vi "StateMachineSubpanel.vi"() -> ()   [LabVIEW 2016]
uses:
  Controls/Config.ctl
  Utilities/DataShare/DataShare.lvclass
  Controls/DAQ.ctl
  Utilities/ControlValues/ControlValues.lvclass
  <vilib>/Utility/error.llb/DialogType.ctl
panel:
  in  "SelectPanel":i32(listbox)=-1
  out "Status":string
  # "Logo"
  # "Blank area for constantly available displays"
  # "Blank area for constantly\navailable displays"
  # "Blank area for constantly available displays, delete splitter if not needed"
  # "Blank area for constantly available displays"
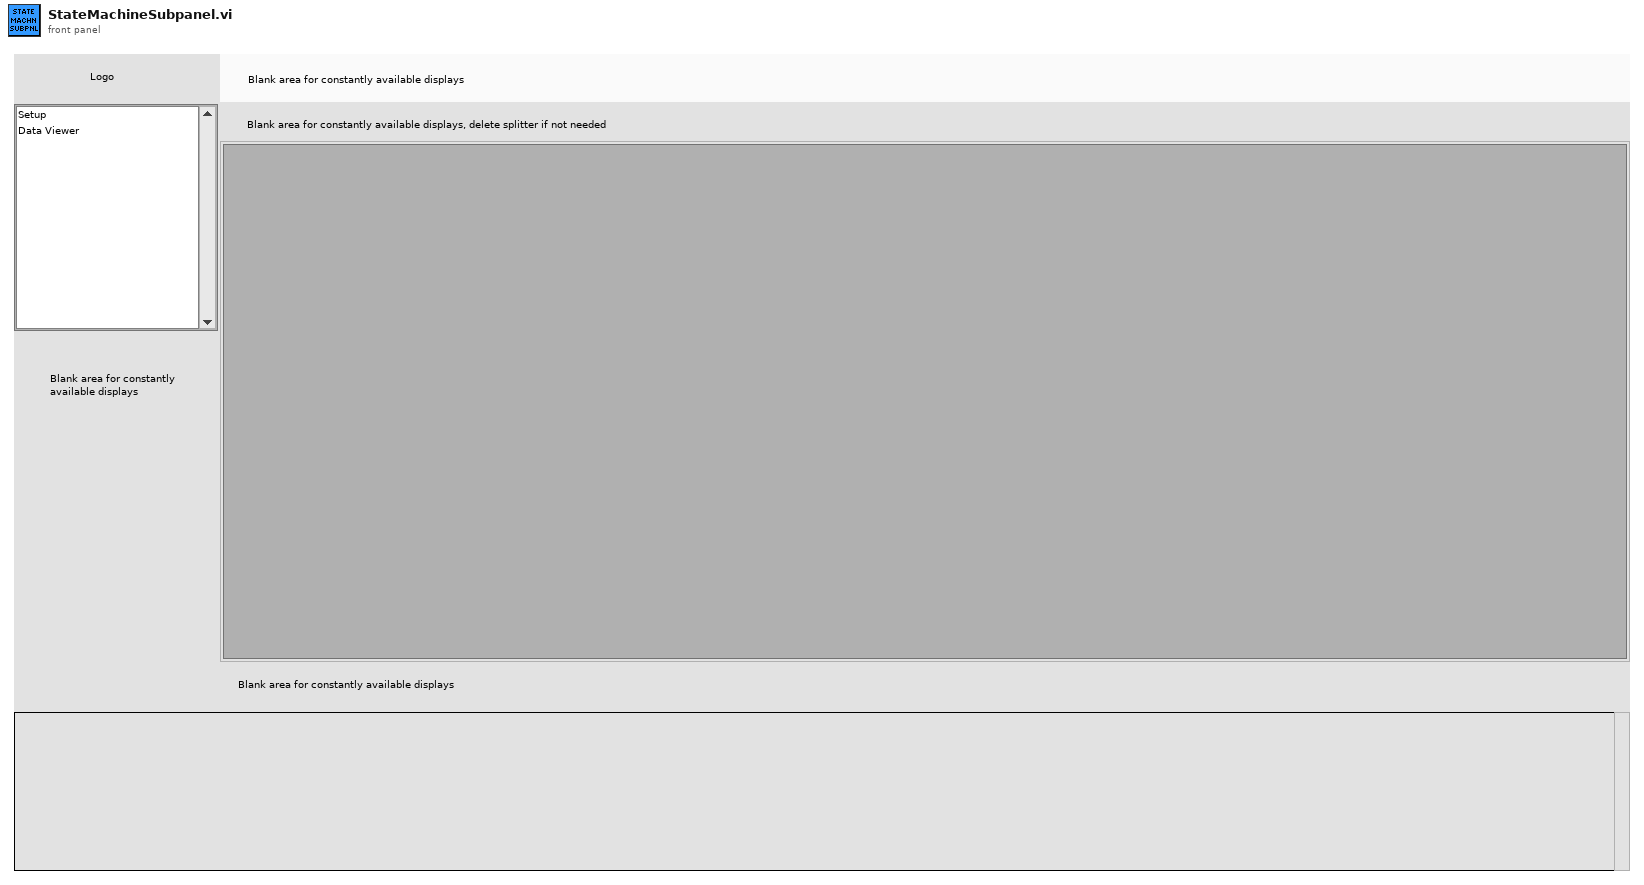
[diagram p1: front panel]
types:
  T1 = typedef "Config.ctl" = cluster{"Subpanels":cluster{"Name":string, "Pathname":string}[], "DAQ":cluster{"Name":string, "Value":string}[]}
  T2 = cluster{"Error":errorcluster, "SubpanelRefs":refnum<vi>[], "SubpanelRef":refnum<vi>, "ControlValues":refnum<class "ControlValues.lvclass">, "AppKind":enum32{"invalid app kind", "Development System", "Run Time System", "Student Edition", "Embedded LabVIEW", "Evaluation", "Custom"}, "LogFolder":path, "ConfigFolder":path, "Config":T1}
  T3 = enum32{"invalid app kind", "Development System", "Run Time System", "Student Edition", "Embedded LabVIEW", "Evaluation", "Custom"}
  T4 = typedef "DialogType.ctl" = u16
  T5 = cluster{"Error":errorcluster, "Config":T1, "Names":string[], "Values":dbl[], "DataShare":refnum<class "DataShare.lvclass">}
  T6 = typedef "DAQ.ctl" = cluster{"Names":string[], "Values":dbl[]}
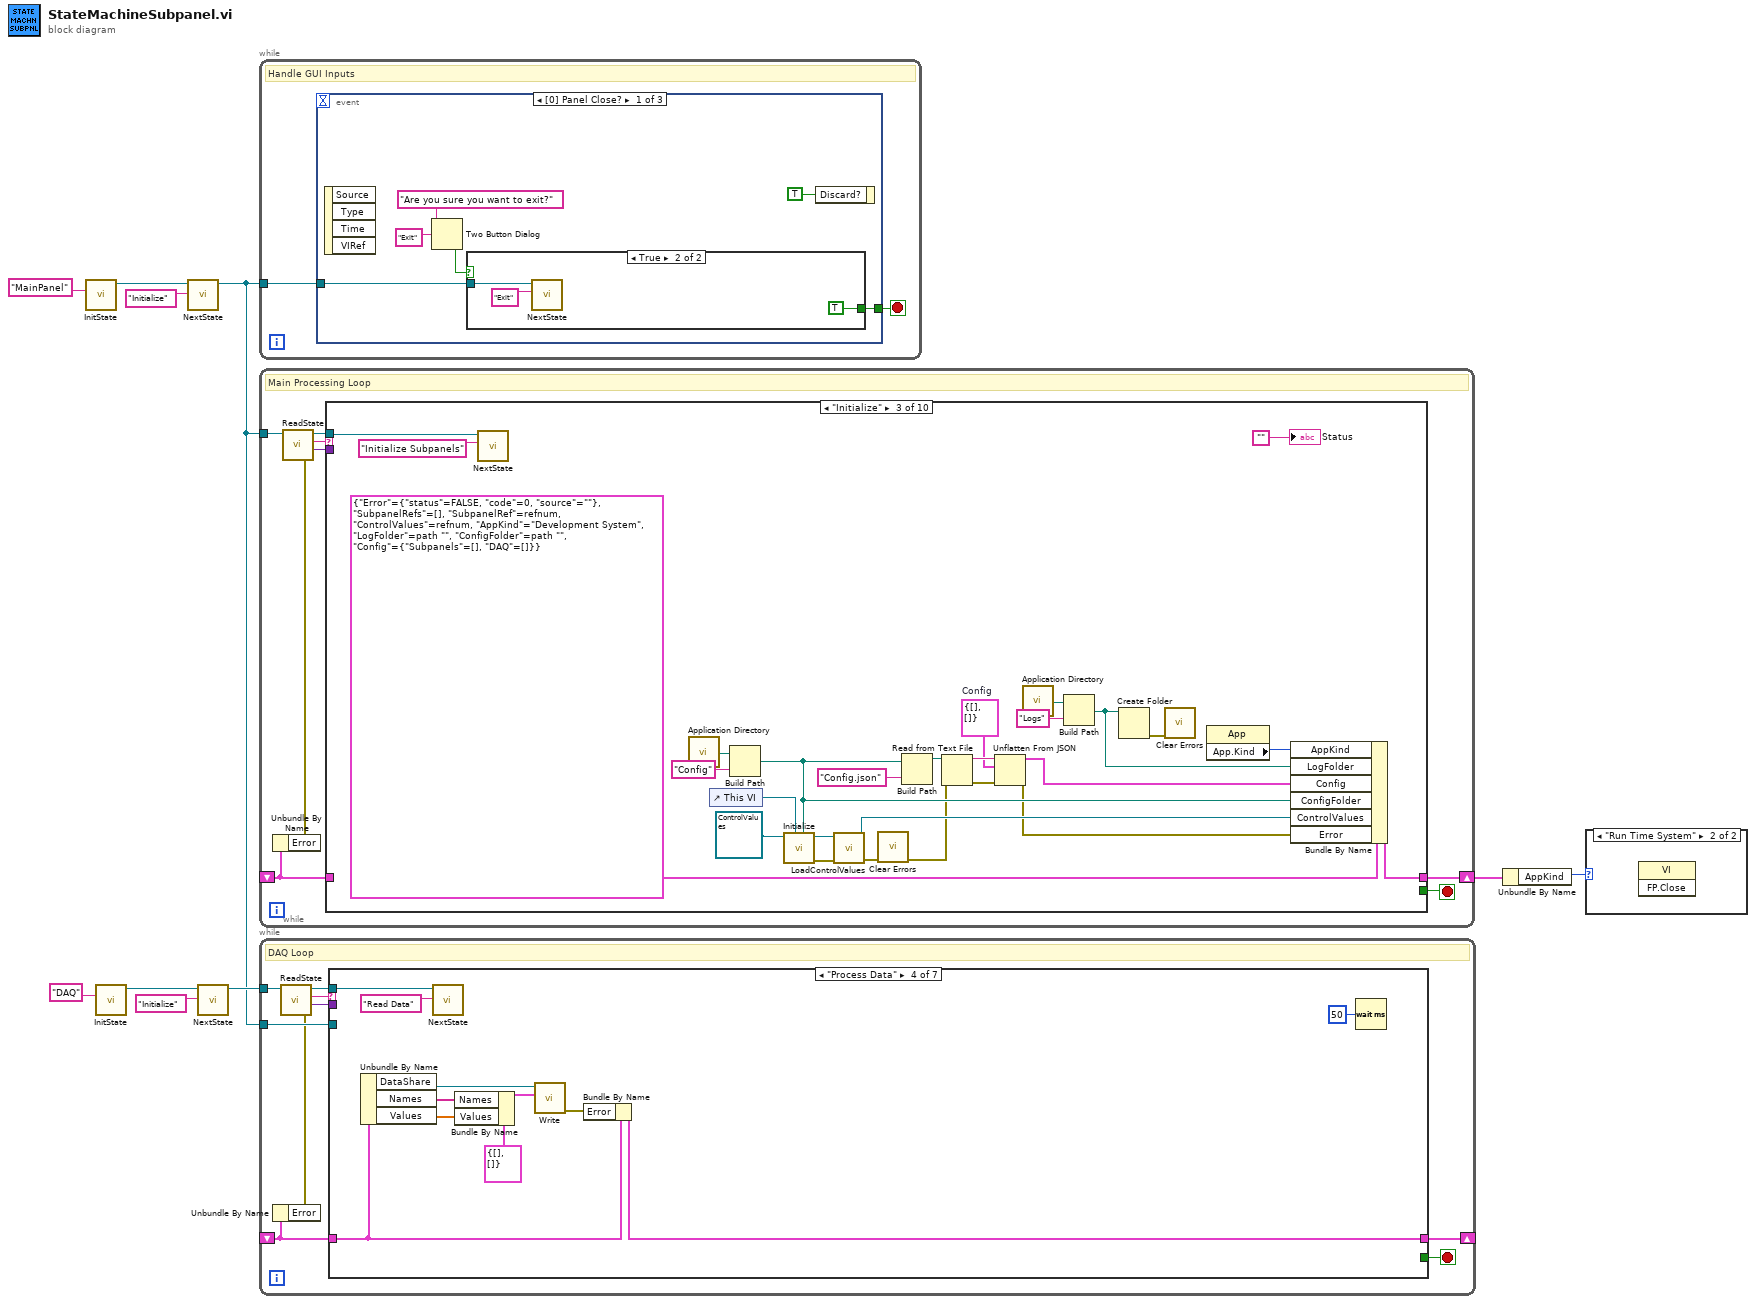
[diagram p0: block diagram]
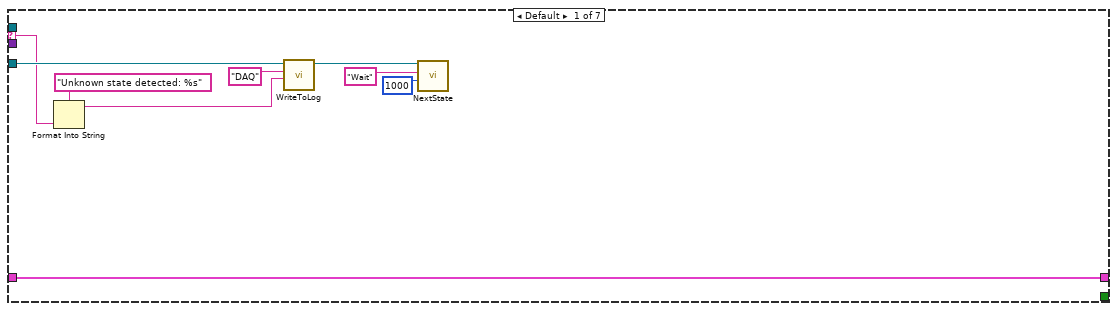
[diagram p2: hidden frame]
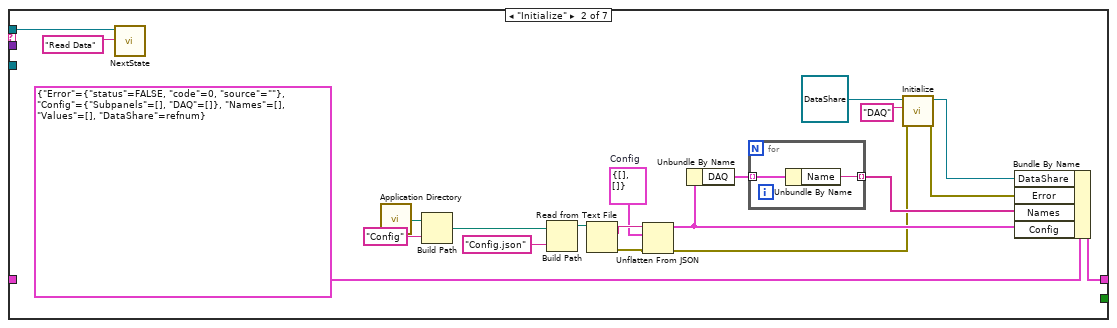
[diagram p3: hidden frame]
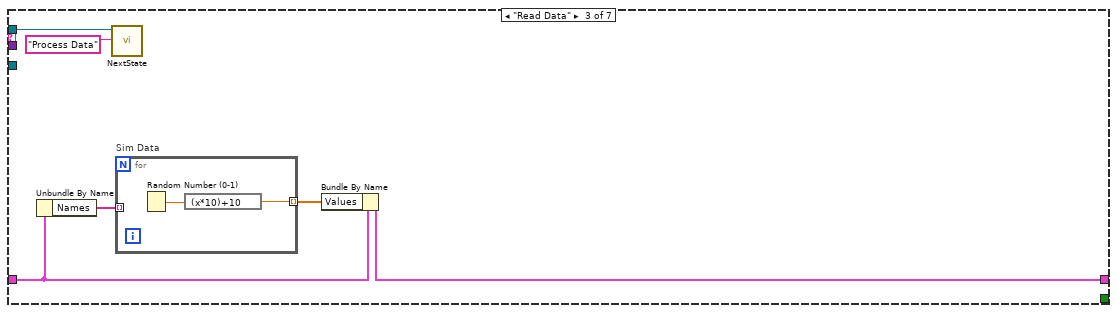
[diagram p4: hidden frame]
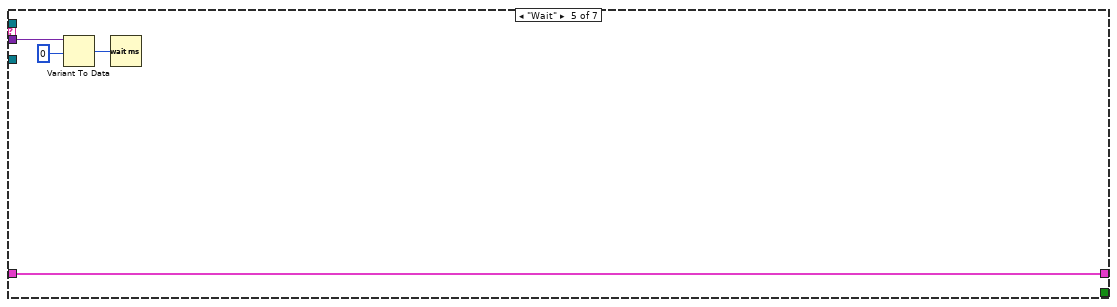
[diagram p5: hidden frame]
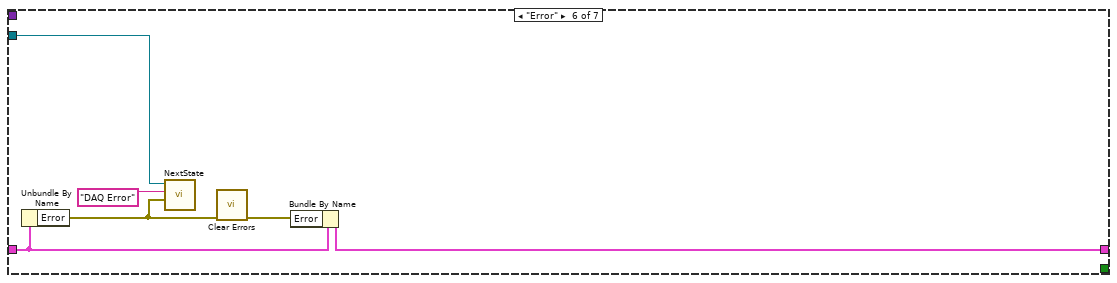
[diagram p6: hidden frame]
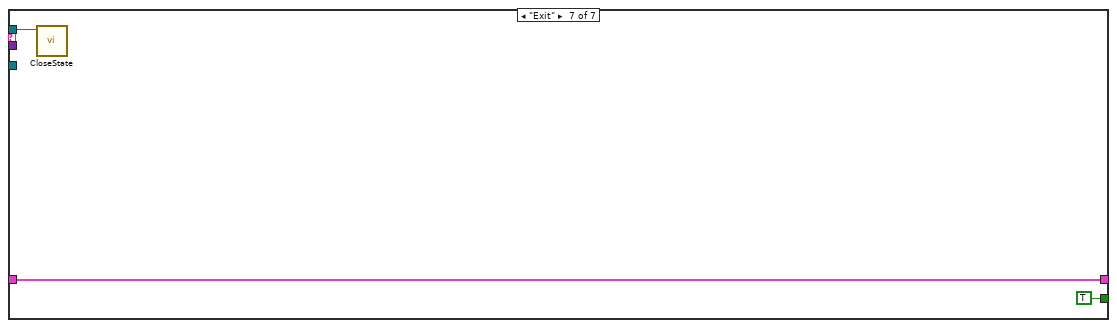
[diagram p7: hidden frame]
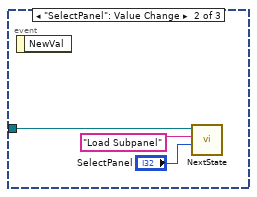
[diagram p10: hidden frame]
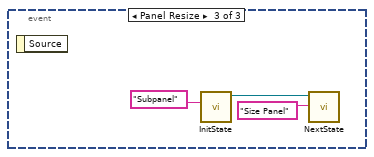
[diagram p11: hidden frame]
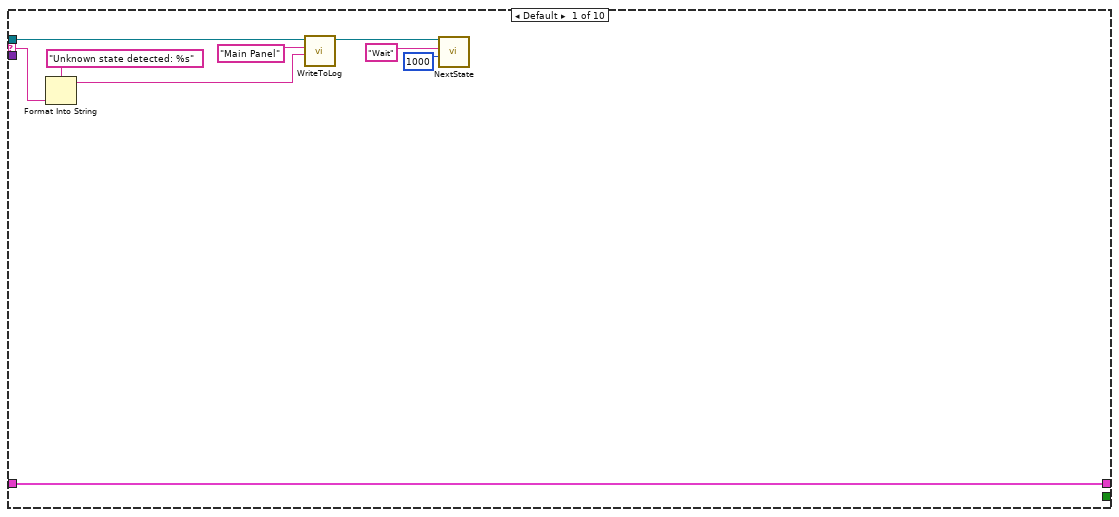
[diagram p12: hidden frame]
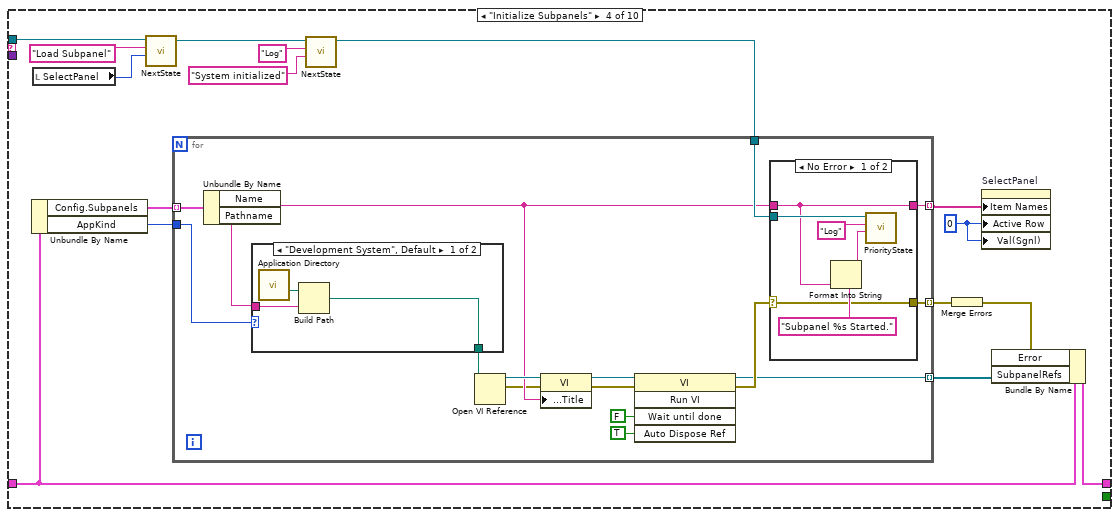
[diagram p14: hidden frame]
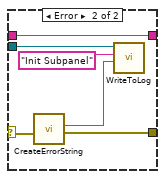
[diagram p15: hidden frame]
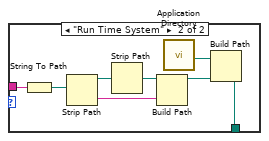
[diagram p16: hidden frame]
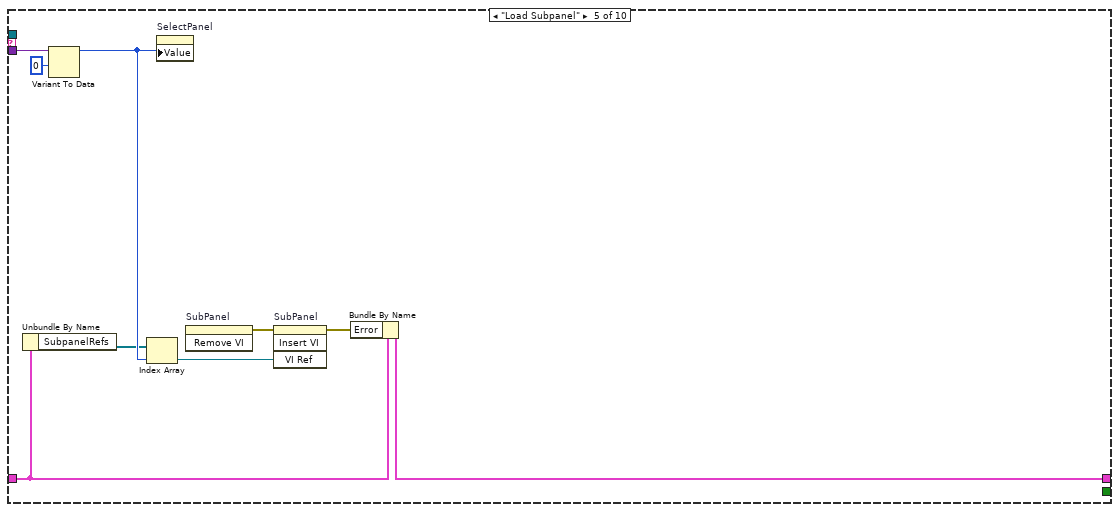
[diagram p17: hidden frame]
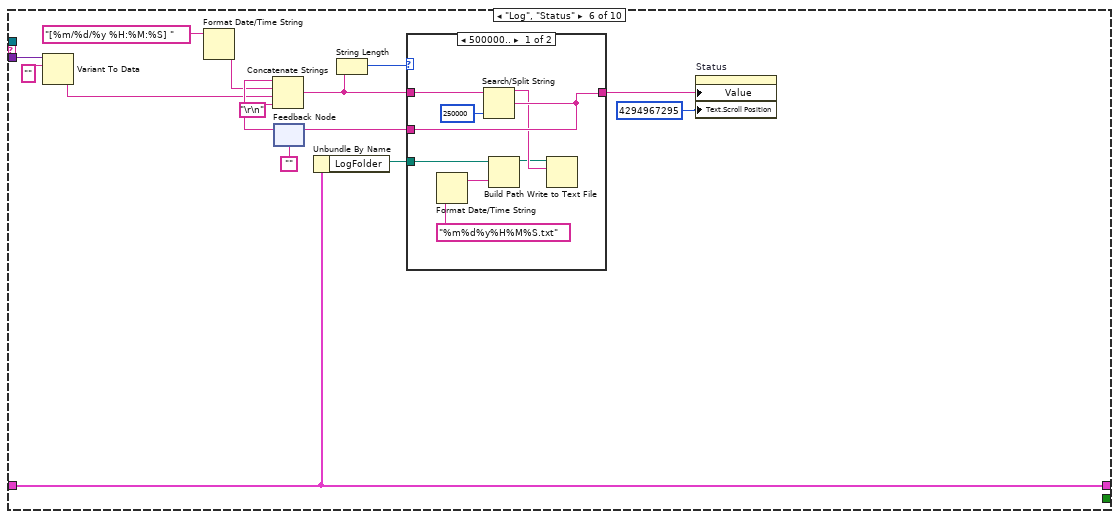
[diagram p18: hidden frame]
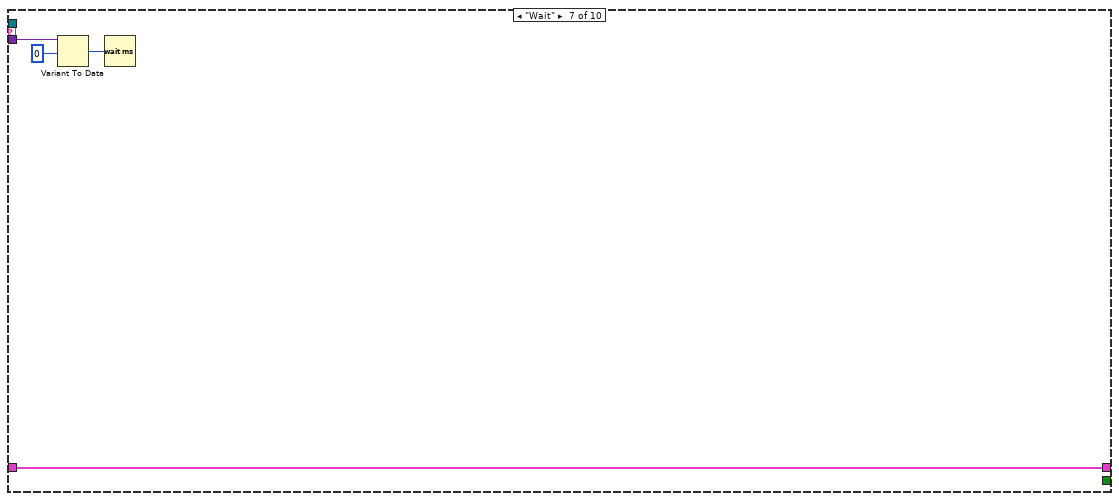
[diagram p20: hidden frame]
diagram:
  n1 = call "InitState.vi"("Name"="MainPanel" ("name (unnamed)")) -> ("Queue Out"=w6:refnum<queue>)  [unwired: 8 in, 1 out]
  n2 = call "InitState.vi"("Name"="DAQ" ("name (unnamed)")) -> ("Queue Out"=w3:refnum<queue>)  [unwired: 8 in, 1 out]
  n3 = call "NextState.vi"("State"="Initialize" ("element"), "Queue In"=w6) -> ("Queue Out"=w1:refnum<queue>)  [unwired: 8 in, 1 out]
  n4 = call "NextState.vi"("State"="Initialize" ("element"), "Queue In"=w3) -> ("Queue Out"=w2:refnum<queue>)  [unwired: 8 in, 1 out]
  n5 = while {
    tunnel: w1 -> [w12]
    stop <- w11 stop-if-true
    # "Handle GUI Inputs"
    n6 = event shown="[0] Panel Close?" {
      selector: _ -> [_ _ _]
      dyn-events: _ -> [_ _ _]
      timeout: _ -> [_ _ _]
      tunnel: w12 -> [w18 w23 _]
      tunnel: [w13 _ _] -> w11
      event Panel Close? {
        n7 = event-data() -> ()  [unwired: 1 in, 4 out]
        n8 = Two Button Dialog(message="Are you sure you want to exit?", 2:"Exit" ("T button name (\"OK\")")) -> (T button?=w14:bool)  [unwired: 1 in]
        n9 = case shown="True" w14 {
          tunnel: w18 -> [_ w19]
          tunnel: [_ TRUE] -> w13
          frame False {
          }
          frame True {
            n10 = call "NextState.vi"("State"="Exit" ("element"), "Queue In"=w19) -> ()  [unwired: 8 in, 2 out]
          }
        }
        n11 = event-data("Discard?"=TRUE) -> ()  [unwired: 1 in, 1 out]
      }
      event "SelectPanel": Value Change {
        n12 = event-data() -> ()  [unwired: 1 in, 1 out]
        n13 = call "NextState.vi"("Data"="SelectPanel", "State"="Load Subpanel", "Queue In"=w23) -> ()  [unwired: 7 in, 2 out]
      }
      event Panel Resize {
        n14 = event-data() -> ()  [unwired: 1 in, 1 out]
        n15 = call "InitState.vi"("Name"="Subpanel" ("name (unnamed)")) -> ("Queue Out"=w25:refnum<queue>)  [unwired: 8 in, 1 out]
        n16 = call "NextState.vi"("State"="Size Panel" ("element"), "Queue In"=w25) -> ()  [unwired: 8 in, 2 out]
      }
    }
  }
  n17 = while {
    tunnel: w1 -> [w33]
    shift-right: [w35] -> w10
    shift-left: _ -> [w29]
    stop <- w34 stop-if-true
    # "Main Processing Loop"
    n18 = Unbundle By Name(w29) -> ("Error"=w28:errorcluster)
    n19 = call "ReadState.vi"("Error In"=w28, "Queue In"=w33) -> ("Data"=w30:variant, "State"=w31:string, "Queue Out"=w32:refnum<queue>)  [unwired: 6 in, 1 out]
    n20 = case shown="\"Initialize\"" w31 {
      tunnel: w32 -> [w41 _ w47 w79 _ _ _ w181 w205 _]
      tunnel: w30 -> [_ _ _ _ w135 w151 w164 w167 _ _]
      selector: w31 -> [w43 _ _ _ _ _ _ w168 _ _]
      tunnel: [w42 w45 w72 w75 w133 w138 w161 w183 w204 w215] -> w35
      tunnel: [_ _ _ _ _ _ _ _ TRUE _] -> w34
      tunnel: w29 -> [w42 w45 _ w76 w132 w138 w161 w166 w204 w215]
      frame Default {
        n21 = Format Into String(format string="Unknown state detected: %s", w43) -> (resulting string=w36:string)  [unwired: 2 in, 1 out]
        n22 = call "WriteToLog.vi"("Data"=w36, "Source"="Main Panel", "Queue In"=w41) -> ("Queue Out"=w40:refnum<queue>)  [unwired: 7 in, 1 out]
        n23 = call "NextState.vi"("Data"=u32 1000, "State"="Wait", "Queue In"=w40) -> ()  [unwired: 7 in, 2 out]
      }
      frame "--- System ---" {
      }
      frame "Initialize" {
        w51 = T1 {"Subpanels"=[], "DAQ"=[]}  # Config
        n24 = call "NextState.vi"("State"="Initialize Subpanels" ("element"), "Queue In"=w47) -> ()  [unwired: 8 in, 2 out]
        n25 = call <vilib>:"Application Directory.vi"() -> ("Application Directory"=w60:path)
        n26 = control-ref of="This VI"() -> (w67:refnum<vi>)
        n27 = Build Path(base path=w60, name or relative path="Config") -> (appended path=w55:path)
        n28 = call "Initialize.vi"("Config Path"=w55, "VI Reference"=w67, "ControlValues in"=refnum<class "ControlValues.lvclass"> refnum) -> ("error out"=w69:errorcluster, "ControlValues out"=w70:refnum<class "ControlValues.lvclass">)  [unwired: 7 in]
        n29 = call "LoadControlValues.vi"("error in"=w69, "ControlValues in"=w70) -> ("error out"=w62:errorcluster, "ControlValues out"=w68:refnum<class "ControlValues.lvclass">)  [unwired: 8 in]
        n30 = call <vilib>:"Clear Errors.vi"("error in (no error)"=w62) -> ("error out"=w52:errorcluster)  [unwired: 5 in, 1 out]
        n31 = Build Path(base path=w55, name or relative path="Config.json") -> (appended path=w56:path)
        n32 = Read from Text File(file (use dialog)=w56, error in=w52) -> (text=w57:string, error out=w58:errorcluster)  [unwired: 2 in, 2 out]
        n33 = Unflatten From JSON(JSON string=w57, type and defaults=w51, error in (no error)=w58) -> (value=w50:T1, error out=w48:errorcluster)  [unwired: 4 in]
        n34 = call <vilib>:"Application Directory.vi"() -> ("Application Directory"=w65:path)
        n35 = Build Path(base path=w65, name or relative path="Logs") -> (appended path=w54:path)
        n36 = Create Folder(path (use dialog)=w54) -> (error out=w63:errorcluster)  [unwired: 2 in, 2 out]
        n37 = call <vilib>:"Clear Errors.vi"("error in (no error)"=w63) -> ()  [unwired: 5 in, 2 out]
        n38 = property class="App"() -> ("App.Kind"=w49:T3)  [unwired: 2 in, 2 out]
        n39 = Bundle By Name(cluster=T2 {"Error"={"status"=FALSE, "code"=0, "source"=""}, "SubpanelRefs"=[], "SubpanelRef"=refnum, "ControlValues"=refnum, "AppKind"=enum."Development System", "LogFolder"=path "", "ConfigFolder"=path "", "Config"={"Subpanels"=[], "DAQ"=[]}}, "AppKind"=w49, "LogFolder"=w54, "Config"=w50, "ConfigFolder"=w55, "ControlValues"=w68, "Error"=w48) -> (w72:T2)
        "Status" <- ""
      }
      frame "Initialize Subpanels" {
        w86 = 0 ("Active Row:Active Row Number")
        n40 = Unbundle By Name(w76) -> ("Config.Subpanels"=w88:cluster{"Name":string, "Pathname":string}[], "AppKind"=w87:T3)
        n41 = local read "SelectPanel"() -> (w83:i32)
        n42 = call "NextState.vi"("Data"=w83, "State"="Load Subpanel" ("element"), "Queue In"=w79) -> ("Queue Out"=w80:refnum<queue>)  [unwired: 7 in, 1 out]
        n43 = call "NextState.vi"("Data"="System initialized" ("State"), "State"="Log", "Queue In"=w80) -> ("Queue Out"=w78:refnum<queue>)  [unwired: 7 in, 1 out]
        n44 = for {
          tunnel: w88 -> [w104] mode=indexing
          tunnel: w87 -> [w102]
          tunnel: w78 -> [w101]
          tunnel: [w96] -> w85 mode=indexing
          tunnel: [w95] -> w77 mode=indexing
          tunnel: [w89] -> w74 mode=indexing
          n45 = Unbundle By Name(w104) -> ("Name"=w93:string, "Pathname"=w103:string)
          n46 = case shown="\"Development System\", Default" w102 {
            tunnel: w103 -> [w118 w127]
            tunnel: [w117 w121] -> w100
            frame "Development System", Default {
              n47 = call <vilib>:"Application Directory.vi"() -> ("Application Directory"=w119:path)
              n48 = Build Path(base path=w119, name or relative path=w118) -> (appended path=w117:path)
            }
            frame "Run Time System" {
              n49 = String To Path(string=w127) -> (path=w126:path)
              n50 = Strip Path(path=w126) -> (stripped path=w125:path, name=w124:string)
              n51 = Strip Path(path=w125) -> (stripped path=w123:path)  [unwired: 1 out]
              n52 = Build Path(base path=w123, name or relative path=w124) -> (appended path=w122:path)
              n53 = call <vilib>:"Application Directory.vi"() -> ("Application Directory"=w120:path)
              n54 = Build Path(base path=w120, name or relative path=w122) -> (appended path=w121:path)
            }
          }
          n55 = Open VI Reference(vi path=w100) -> (vi reference=w94:refnum<vi>, error out=w90:errorcluster)  [unwired: 5 in]
          n56 = property class="VI"(reference=w94, error in=w90, "Front Panel.Title"=w93) -> (reference out=w92:refnum<vi>, error out=w91:errorcluster)
          n57 = invoke class="VI" method="Run VI"(reference=w92, error in=w91, "Wait until done"=FALSE ("Wait Until Done"), "Auto Dispose Ref"=TRUE ("Auto Dispose Reference")) -> (reference out=w95:refnum<vi>, error out=w97:errorcluster)  [unwired: 1 in, 3 out]
          n58 = case shown="No Error" w97 {
            selector: w97 -> [w105 w115]
            tunnel: w101 -> [w109 w114]
            tunnel: w93 -> [w106 w116]
            tunnel: [w106 w116] -> w96
            tunnel: [w105 w111] -> w89
            frame No Error {
              n59 = Format Into String(format string="Subpanel %s Started.", w106) -> (resulting string=w107:string)  [unwired: 2 in, 1 out]
              n60 = call "PriorityState.vi"("Data"=w107, "State"="Log" ("element"), "Queue In"=w109) -> ()  [unwired: 7 in, 2 out]
            }
            frame Error {
              n61 = call "CreateErrorString.vi"("Error In"=w115) -> ("Error Out"=w111:errorcluster, "Error String"=w112:string)  [unwired: 9 in]
              n62 = call "WriteToLog.vi"("Data"=w112, "Source"="Init Subpanel", "Queue In"=w114) -> ()  [unwired: 7 in, 2 out]
            }
          }
        }
        n63 = Merge Errors(w74) -> (w73:errorcluster)
        n64 = property on="SelectPanel" class="LstBox (strict)"("Item Names"=w85, "Active Row"=w86, "Val(Sgnl)"=w86) -> ()  [unwired: 2 in, 2 out]
        n65 = Bundle By Name(cluster=w76, "Error"=w73, "SubpanelRefs"=w77) -> (w75:T2)
      }
      frame "Load Subpanel" {
        n66 = Unbundle By Name(w132) -> ("SubpanelRefs"=w129:refnum<vi>[])
        n67 = Variant To Data(type=0, Variant=w135) -> (data=w130:i32)  [unwired: 1 in, 1 out]
        n68 = Index Array(array=w129, index=w130) -> (element=w128:refnum<vi>)
        n69 = property on="SelectPanel" class="LstBox (strict)"("Value"=w130) -> ()  [unwired: 2 in, 2 out]
        n70 = invoke on="SubPanel" class="SubPnl" method="Remove VI"() -> (error out=w134:errorcluster)  [unwired: 3 in, 2 out]
        n71 = invoke on="SubPanel" class="SubPnl" method="Insert VI"(error in=w134, "VI Ref"=w128) -> (error out=w131:errorcluster)  [unwired: 2 in, 3 out]
        n72 = Bundle By Name(cluster=w132, "Error"=w131) -> (w133:T2)
      }
      frame "Log", "Status" {
        n73 = Variant To Data(type="", Variant=w151) -> (data=w144:string)  [unwired: 1 in, 1 out]
        n74 = Format Date/Time String(time format string (%c)="[%m/%d/%y %H:%M:%S] ") -> (date/time string=w145:string)  [unwired: 2 in]
        n75 = feedback #1("") -> (w147:string)
        n76 = Concatenate Strings(w147, w145, w144, "\r\n") -> (w141:string)
        n77 = Unbundle By Name(w138) -> ("LogFolder"=w137:path)
        n78 = String Length(string=w141) -> (length=w142:i32)
        n79 = case shown="500000.." w142 {
          tunnel: [w157 w160] -> w140
          tunnel: w141 -> [w159 w160]
          tunnel: [w157 w160] -> w139
          tunnel: w137 -> [w154 _]
          frame 500000.. {
            n80 = Format Date/Time String(time format string (%c)="%m%d%y%H%M%S.txt" ("name or relative path")) -> (date/time string=w155:string)  [unwired: 2 in]
            n81 = Search/Split String(string=w159, offset (0)=250000) -> (substring before match=w156:string, match + rest of string=w157:string)  [unwired: 1 in, 1 out]
            n82 = Build Path(base path=w154, name or relative path=w155) -> (appended path=w153:path)
            n83 = Write to Text File(file (use dialog)=w153, text=w156) -> ()  [unwired: 2 in, 3 out]
          }
          frame Default {
          }
        }
        n84 = feedback-in #1(w139) -> ()
        n85 = property on="Status" class="Str"("Value"=w140, "Text.Scroll Position"=u32 4294967295) -> ()  [unwired: 2 in, 2 out]
      }
      frame "Wait" {
        n86 = Variant To Data(type=u32 0, Variant=w164) -> (data=w162:u32)  [unwired: 1 in, 1 out]
        n87 = Wait (ms)(milliseconds to wait=w162) -> ()  [unwired: 1 out]
      }
      frame "DAQ Error", "Error" {
        w175 = T4 0 items=["no dialog", "OK message", "continue or stop message", "OK message + warnings", "continue/stop + warnings"] ("type of dialog (OK msg:1)")
        n88 = case shown="\"DAQ Error\"" w168 {
          tunnel: w167 -> [_ w188]
          tunnel: w166 -> [w185 _]
          tunnel: [w184 w186] -> w165
          frame Default {
            n89 = Unbundle By Name(w185) -> ("Error"=w184:errorcluster)
          }
          frame "DAQ Error" {
            n90 = Variant To Data(type=errorcluster {"status"=FALSE, "code"=0, "source"=""} ("Error"), Variant=w188) -> (data=w186:errorcluster)  [unwired: 1 in, 1 out]
          }
        }
        n91 = call <vilib>:"General Error Handler.vi"("search ni.com link visible?(T)"=FALSE, "type of dialog (OK msg:1)"=w175, "error in (no error)"=w165) -> ("message"=w172:string, "error out"=w176:errorcluster)  [unwired: 8 in, 3 out]
        n92 = call <vilib>:"Clear Errors.vi"("error in (no error)"=w176) -> ("error out"=w182:errorcluster)  [unwired: 5 in, 1 out]
        n93 = call "FlushState.vi"("Queue In"=w181) -> ("Queue Out"=w180:refnum<queue>)  [unwired: 9 in, 1 out]
        n94 = Search and Replace String(replace all?=TRUE ("replace all? (F)"), input string=w172, search string="\r\n", replace string=" " ("replace string (\"\")")) -> (result string=w173:string)  [unwired: 4 in, 3 out]
        n95 = Bundle By Name(cluster=w166, "Error"=w182) -> (w183:T2)
        n96 = Format Into String(format string="[ERROR] %s", w173) -> (resulting string=w177:string)  [unwired: 2 in, 1 out]
        n97 = call "NextState.vi"("Data"=w177, "State"="Log" ("element"), "Queue In"=w180) -> ()  [unwired: 7 in, 2 out]
      }
      frame "Exit" {
        n98 = Unbundle By Name(w204) -> ("Config.Subpanels"=w192:cluster{"Name":string, "Pathname":string}[], "ControlValues"=w203:refnum<class "ControlValues.lvclass">, "LogFolder"=w195:path)
        n99 = call "CloseState.vi"("Queue In"=w205) -> ()  [unwired: 10 in, 1 out]
        n100 = invoke on="SubPanel" class="SubPnl" method="Remove VI"() -> (error out=w193:errorcluster)  [unwired: 3 in, 2 out]
        n101 = for {
          tunnel: w193 -> [w209]
          tunnel: w192 -> [w208] mode=indexing
          n102 = Unbundle By Name(w208) -> ("Name"=w207:string)
          n103 = call "InitState.vi"("Error In"=w209, "Name"=w207) -> ("Queue Out"=w210:refnum<queue>)  [unwired: 7 in, 1 out]
          n104 = call "PriorityState.vi"("State"="Exit", "Queue In"=w210) -> ()  [unwired: 8 in, 2 out]
        }
        n105 = Format Date/Time String(time format string (%c)="%m%d%y%H%M%S.txt" ("name or relative path")) -> (date/time string=w199:string)  [unwired: 2 in]
        n106 = Build Path(base path=w195, name or relative path=w199) -> (appended path=w202:path)
        n107 = local read "Status"() -> (w201:string)
        n108 = Write to Text File(file (use dialog)=w202, text=w201) -> (error out=w198:errorcluster)  [unwired: 2 in, 2 out]
        n109 = call <vilib>:"Clear Errors.vi"("error in (no error)"=w198) -> ("error out"=w196:errorcluster)  [unwired: 5 in, 1 out]
        n110 = disable-structure shown="Enabled" {
          disable-tunnel: [w212 w214] -> w197
          disable-tunnel: w196 -> [w212 w214]
          frame Disabled {
          }
          frame Enabled {
            n111 = local write "Status"("") -> ()
          }
        }
        n112 = call "SaveControlValues.vi"("error in"=w197, "ControlValues in"=w203) -> ("error out"=w194:errorcluster)  [unwired: 7 in, 2 out]
        n113 = call <vilib>:"Clear Errors.vi"("error in (no error)"=w194) -> ()  [unwired: 5 in, 2 out]
        n114 = call "InitState.vi"("Name"="DAQ" ("name (unnamed)")) -> ("Queue Out"=w189:refnum<queue>)  [unwired: 8 in, 1 out]
        n115 = call "NextState.vi"("State"="Exit" ("element"), "Queue In"=w189) -> ()  [unwired: 8 in, 2 out]
      }
      frame "--- Add Customizations Here ---" {
      }
    }
  }
  n116 = while {
    tunnel: w2 -> [w224]
    tunnel: w1 -> [w220]
    shift-right: [w218] -> _
    shift-left: _ -> [w217]
    stop <- w219 stop-if-true
    # "DAQ Loop"
    n117 = Unbundle By Name(w217) -> ("Error"=w216:errorcluster)
    n118 = call "ReadState.vi"("Error In"=w216, "Queue In"=w224) -> ("Data"=w221:variant, "State"=w222:string, "Queue Out"=w223:refnum<queue>)  [unwired: 6 in, 1 out]
    n119 = case shown="\"Process Data\"" w222 {
      tunnel: w223 -> [_ w252 w260 w273 _ _ w285]
      tunnel: w221 -> [_ _ _ _ w276 _ _]
      selector: w222 -> [w226 _ _ _ _ _ _]
      tunnel: w220 -> [w227 _ _ _ _ w284 _]
      tunnel: [_ _ _ _ _ _ TRUE] -> w219
      tunnel: [w225 w243 w256 w268 w275 w279 w286] -> w218
      tunnel: w217 -> [w225 _ w257 w269 w275 w280 w286]
      frame Default {
        n120 = Format Into String(format string="Unknown state detected: %s", w226) -> (resulting string=w228:string)  [unwired: 2 in, 1 out]
        n121 = call "WriteToLog.vi"("Data"=w228, "Source"="DAQ", "Queue In"=w227) -> ("Queue Out"=w232:refnum<queue>)  [unwired: 7 in, 1 out]
        n122 = call "NextState.vi"("Data"=u32 1000, "State"="Wait", "Queue In"=w232) -> ()  [unwired: 7 in, 2 out]
      }
      frame "Initialize" {
        w246 = T1 {"Subpanels"=[], "DAQ"=[]}  # Config
        n123 = call "NextState.vi"("State"="Read Data" ("element"), "Queue In"=w252) -> ()  [unwired: 8 in, 2 out]
        n124 = call <vilib>:"Application Directory.vi"() -> ("Application Directory"=w250:path)
        n125 = Build Path(base path=w250, name or relative path="Config") -> (appended path=w248:path)
        n126 = Build Path(base path=w248, name or relative path="Config.json") -> (appended path=w249:path)
        n127 = Read from Text File(file (use dialog)=w249) -> (text=w247:string, error out=w245:errorcluster)  [unwired: 3 in, 2 out]
        n128 = Unflatten From JSON(JSON string=w247, type and defaults=w246, error in (no error)=w245) -> (value=w241:T1, error out=w236:errorcluster)  [unwired: 4 in]
        n129 = Unbundle By Name(w241) -> ("DAQ"=w240:cluster{"Name":string, "Value":string}[])
        n130 = for {
          tunnel: w240 -> [w255] mode=indexing
          tunnel: [w254] -> w239 mode=indexing
          n131 = Unbundle By Name(w255) -> ("Name"=w254:string)
        }
        n132 = call "Initialize.vi"("error in (no error)"=w236, "Name"="DAQ", "DataShare in"=refnum<class "DataShare.lvclass"> refnum) -> ("error out"=w235:errorcluster, "DataShare out"=w234:refnum<class "DataShare.lvclass">)  [unwired: 7 in]
        n133 = Bundle By Name(cluster=T5 {"Error"={"status"=FALSE, "code"=0, "source"=""}, "Config"={"Subpanels"=[], "DAQ"=[]}, "Names"=[], "Values"=[], "DataShare"=refnum}, "DataShare"=w234, "Error"=w235, "Names"=w239, "Config"=w241) -> (w243:T5)
      }
      frame "Read Data" {
        n134 = Unbundle By Name(w257) -> ("Names"=w259:string[])
        n135 = call "NextState.vi"("State"="Process Data" ("element"), "Queue In"=w260) -> ()  [unwired: 8 in, 2 out]
        n136 = for "Sim Data" {
          tunnel: w259 -> [_] mode=indexing
          tunnel: [w262] -> w258 mode=indexing
          n137 = Random Number (0-1)() -> (number: 0 to 1=w263:dbl)
          n138 = expression code="(x*10)+10"(w263) -> (w262:dbl)
        }
        n139 = Bundle By Name(cluster=w257, "Values"=w258) -> (w256:T5)
      }
      frame "Process Data" {
        n140 = Unbundle By Name(w269) -> ("DataShare"=w271:refnum<class "DataShare.lvclass">, "Names"=w266:string[], "Values"=w265:dbl[])
        n141 = call "NextState.vi"("State"="Read Data" ("element"), "Queue In"=w273) -> ()  [unwired: 8 in, 2 out]
        n142 = Bundle By Name(cluster=T6 {"Names"=[], "Values"=[]} ("DAQ"), "Names"=w266, "Values"=w265) -> (w264:T6)
        n143 = call "Write.vi"("Data"=w264, "DataShare in"=w271) -> ("error out"=w270:errorcluster)  [unwired: 8 in, 1 out]
        n144 = Bundle By Name(cluster=w269, "Error"=w270) -> (w268:T5)
        n145 = Wait (ms)(milliseconds to wait=u32 50) -> ()  [unwired: 1 out]
      }
      frame "Wait" {
        n146 = Variant To Data(type=u32 0, Variant=w276) -> (data=w278:u32)  [unwired: 1 in, 1 out]
        n147 = Wait (ms)(milliseconds to wait=w278) -> ()  [unwired: 1 out]
      }
      frame "Error" {
        n148 = Unbundle By Name(w280) -> ("Error"=w282:errorcluster)
        n149 = call "NextState.vi"("Data"=w282, "State"="DAQ Error", "Queue In"=w284) -> ()  [unwired: 7 in, 2 out]
        n150 = call <vilib>:"Clear Errors.vi"("error in (no error)"=w282) -> ("error out"=w281:errorcluster)  [unwired: 5 in, 1 out]
        n151 = Bundle By Name(cluster=w280, "Error"=w281) -> (w279:T5)
      }
      frame "Exit" {
        n152 = call "CloseState.vi"("Queue In"=w285) -> ()  [unwired: 10 in, 1 out]
      }
    }
  }
  n153 = Unbundle By Name(w10) -> ("AppKind"=w7:T3)
  n154 = case shown="\"Run Time System\"" w7 {
    frame Default {
    }
    frame "Run Time System" {
      n155 = invoke class="VI" method="FP.Close"() -> ()  [unwired: 3 in, 3 out]
    }
  }
